vi "updateTimer.vi"(8 "error in (no error)":errorcluster, 11 "SpectrographHeartbeat in":refnum<class "SpectrographHeartbeat.lvclass">) -> (0 "error out":errorcluster, 2 "getStatus?":bool, 3 "SpectrographHeartbeat out":refnum<class "SpectrographHeartbeat.lvclass">)   [LabVIEW 2016, in "SpectrographHeartbeat.lvclass"]
uses:
  SpectrographHeartbeat.lvclass
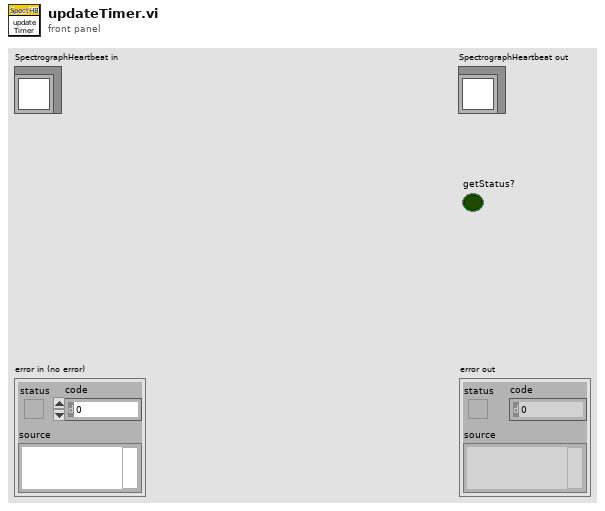
[diagram p1: front panel]
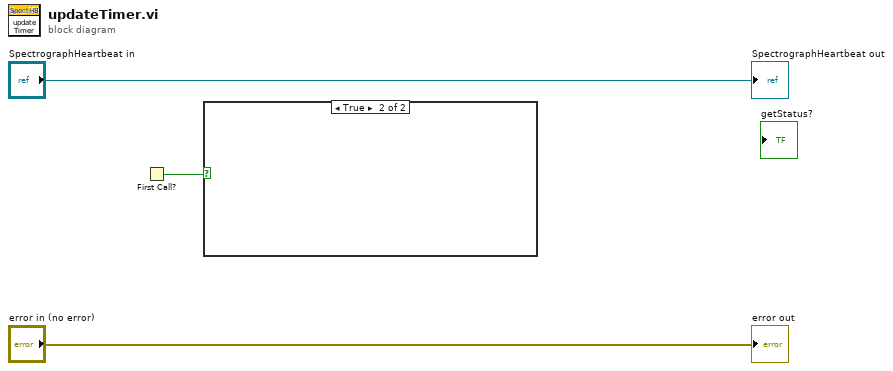
[diagram p0: block diagram]
diagram:
  n1 = First Call?() -> (First Call?: T/F=w1:bool)
  n2 = case shown="True" w1 {
    frame False {
    }
    frame True {
    }
  }
  "error out" <- "error in (no error)"
  "SpectrographHeartbeat out" <- "SpectrographHeartbeat in"
